vi "Strain Configure 4Wire.vi"(5 "ChannelList":string, 6 "Resolution":dbl, 7 "Range":dbl, 8 "error in (no error)":errorcluster {"code" format="%.0x"}, 9 "GaugeFactor":dbl, 10 "GaugeResistance":dbl, 11 "instrument handle":refnum<k15>) -> (0 "error out":errorcluster {"code" format="%.0x"}, 3 "instrument handle out":refnum<k15>)   [LabVIEW 2020, in "Keysight DAQ970.lvlib"]
doc: "Configures the specified channels for direct 4-wire strain gauge measurement, but does not initiate a scan. This command redefines the scan list."
uses:
  Keysight DAQ970.lvlib
  KtDAQ970.dll
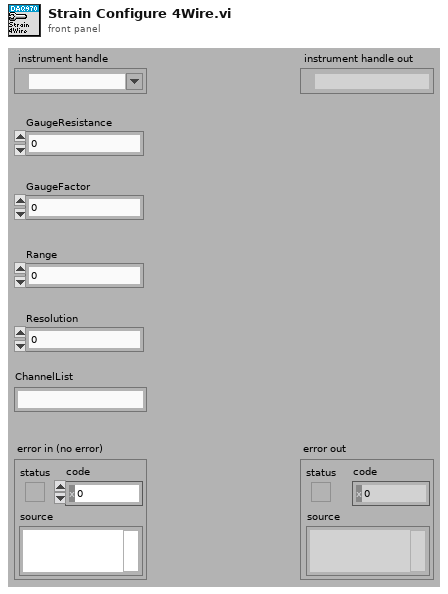
[diagram p1: front panel]
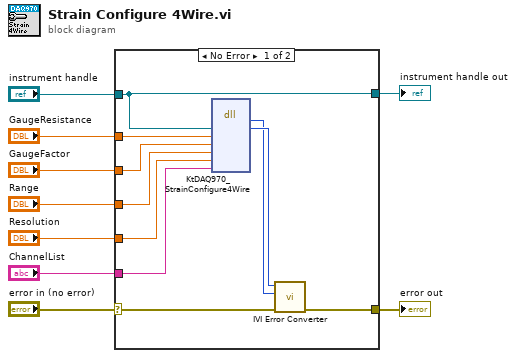
[diagram p0: block diagram]
diagram:
  n1 = case shown="No Error" "error in (no error)" {
    selector: "error in (no error)" -> [w17 w21]
    tunnel: [w16 w21] -> w9
    tunnel: "instrument handle" -> [w10 w20]
    tunnel: "GaugeResistance" -> [w15 _]
    tunnel: "GaugeFactor" -> [w14 _]
    tunnel: "Range" -> [w13 _]
    tunnel: "Resolution" -> [w12 _]
    tunnel: "ChannelList" -> [w11 _]
    tunnel: [w10 w20] -> w1
    frame No Error {
      n2 = dll-call lib="KtDAQ970**.dll" fn="KtDAQ970_StrainConfigure4Wire"("Vi"=w10, "GaugeResistance"=w15, "GaugeFactor"=w14, "Range"=w13, "Resolution"=w12, "ChannelList"=w11) -> (w18:i32, "Vi"=w19:u32)  [unwired: 8 in, 2 out]
      n3 = call "IVI Error Converter.vi"("error in (no error)"=w17, "IVI error code (0)"=w18, "instrument handle"=w19) -> ("error out"=w16:errorcluster)  [unwired: 7 in, 1 out]
    }
    frame Error {
    }
  }
  "error out" <- w9
  "instrument handle out" <- w1
